vi "CRYLowUp360to180.vi"(10 "Value In":dbl) -> (2 "Value Out":dbl)   [LabVIEW 2013]
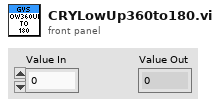
[diagram p1: front panel]
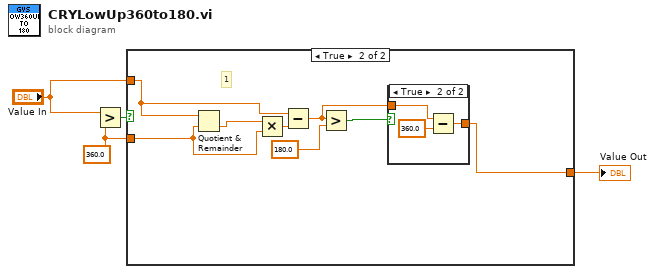
[diagram p0: block diagram]
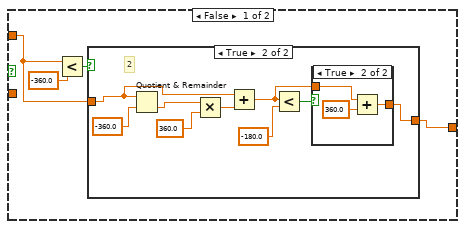
[diagram p2: hidden frame]
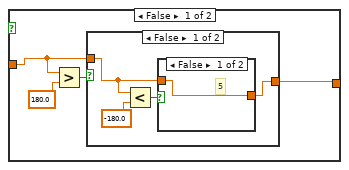
[diagram p3: hidden frame]
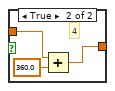
[diagram p4: hidden frame]
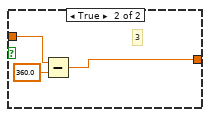
[diagram p5: hidden frame]
diagram:
  w3 = 360.0 ("y")
  n1 = Greater?(x="Value In", y=w3) -> (0:w4:bool)
  n2 = case shown="True" w4 {
    tunnel: "Value In" -> [w6 w42]
    tunnel: w3 -> [_ w44]
    tunnel: [w5 w38] -> w1
    frame False {
      n3 = Less?(x=w6, y=-360.0) -> (x < y?=w8:bool)
      n4 = case shown="True" w8 {
        tunnel: w6 -> [w10 w31]
        tunnel: [w9 w27] -> w5
        frame False {
          n5 = Greater?(x=w10, y=180.0) -> (0:w11:bool)
          n6 = case shown="False" w11 {
            tunnel: w10 -> [w14 w23]
            tunnel: [w13 w21] -> w9
            frame False {
              n7 = Less?(x=w14, y=-180.0) -> (x < y?=w15:bool)
              n8 = case shown="False" w15 {
                tunnel: w14 -> [w17 w20]
                tunnel: [w17 w18] -> w13
                frame False {
                  # "5"
                }
                frame True {
                  # "4"
                  n9 = Add(x=w20, y=360.0) -> (x+y=w18:dbl)
                }
              }
            }
            frame True {
              # "3"
              n10 = Subtract(x=w23, y=360.0) -> (x-y=w21:dbl)
            }
          }
        }
        frame True {
          # "2"
          n11 = Quotient & Remainder(x=w31, y=-360.0) -> (floor(x/y)=w26:dbl)  [unwired: 1 out]
          n12 = Multiply(x=w26, y=360.0) -> (x*y=w32:dbl)
          n13 = Add(x=w31, y=w32) -> (x+y=w28:dbl)
          n14 = Less?(x=w28, y=-180.0) -> (x < y?=w29:bool)
          n15 = case shown="True" w29 {
            tunnel: w28 -> [w33 w36]
            tunnel: [w33 w34] -> w27
            frame False {
            }
            frame True {
              n16 = Add(x=w36, y=360.0) -> (x+y=w34:dbl)
            }
          }
        }
      }
    }
    frame True {
      # "1"
      n17 = Quotient & Remainder(x=w42, y=w44) -> (floor(x/y)=w37:dbl)  [unwired: 1 out]
      n18 = Multiply(x=w37, y=w44) -> (x*y=w43:dbl)
      n19 = Subtract(x=w42, y=w43) -> (x-y=w39:dbl)
      n20 = Greater?(x=w39, y=180.0) -> (0:w40:bool)
      n21 = case shown="True" w40 {
        tunnel: w39 -> [w45 w48]
        tunnel: [w45 w46] -> w38
        frame False {
        }
        frame True {
          n22 = Subtract(x=w48, y=360.0) -> (x-y=w46:dbl)
        }
      }
    }
  }
  "Value Out" <- w1
